vi "Slow Loop Controller.vi"(6 "error in":errorcluster, 7 "Slow Loop State in":T1 {"Phi Setpoint" format="%#_13g"}, 8 "Slow Loop Gains":T2) -> (0 "error out":errorcluster, 1 "Slow Loop State out":T1)   [LabVIEW 2014]
uses:
  <vilib>/ptbypt/NI_PtbyPt.lvlib
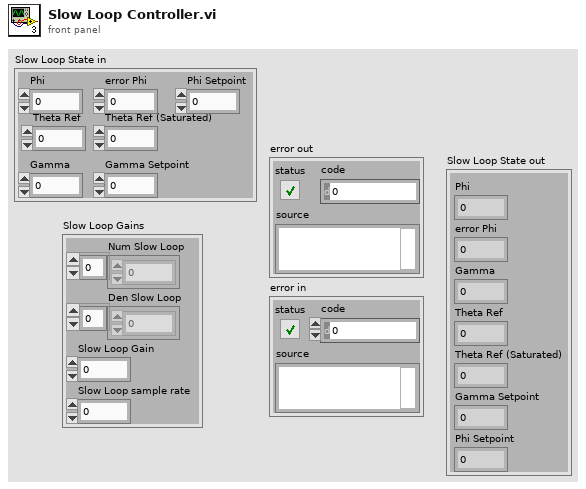
[diagram p1: front panel]
types:
  T1 = cluster{"Phi":dbl, "error Phi":dbl, "Gamma":dbl, "Theta Ref":dbl, "Theta Ref (Saturated)":sgl, "Gamma Setpoint":dbl, "Phi Setpoint":dbl}
  T2 = cluster{"Num Slow Loop":dbl[], "Den Slow Loop":dbl[], "Slow Loop Gain":dbl, "Slow Loop sample rate":dbl}
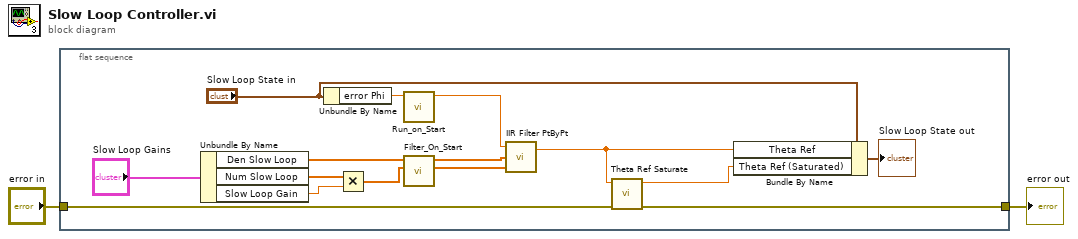
[diagram p0: block diagram]
diagram:
  n1 = flat-sequence {
    tunnel: "error in" -> [w17]
    tunnel: [w16] -> w1
    frame #0 {
      n2 = Unbundle By Name("Slow Loop Gains") -> ("Den Slow Loop"=w5:dbl[], "Num Slow Loop"=w6:dbl[], "Slow Loop Gain"=w11:dbl)
      n3 = Unbundle By Name("Slow Loop State in") -> ("error Phi"=w10:dbl)
      n4 = Multiply(x=w6, y=w11) -> (x*y=w13:dbl[])
      n5 = call "Run_on_Start.vi"("val in"=w10) -> ("Val out"=w9:sgl)  [unwired: 10 in]
      n6 = call "Filter_On_Start.vi"("Num In"=w13, "Denom In"=w5) -> ("Num out"=w14:dbl[], "Denom Out"=w15:dbl[])  [unwired: 8 in]
      n7 = call <vilib>:"IIR Filter PtByPt.vi"("Forward Coefficients"=w14, "Reverse Coefficients"=w15, "x"=w9) -> ("Filtered x"=w8:dbl)  [unwired: 1 in, 1 out]
      n8 = call "Theta Ref Saturate.vi"("error in (no error)"=w17, "Filtered x"=w8) -> ("error out"=w16:errorcluster, "Theta Ref (Saturated)"=w7:sgl)  [unwired: 8 in]
      n9 = Bundle By Name(cluster="Slow Loop State in", "Theta Ref"=w8, "Theta Ref (Saturated)"=w7) -> (→"Slow Loop State out":T1)
    }
  }
  "error out" <- w1
